vi "READ POV angles.vi"(10 "Buttons":bool[](array[boolean]), 11 "POVs":i16[](array[numeric])) -> ()   [LabVIEW 2020]
uses:
  defCameraPOVservos.ctl
  <vilib>/Analysis/coordinate.llb/Angle Range (Degree).ctl
  <vilib>/Analysis/coordinate.llb/Angle Units.ctl
  <vilib>/Analysis/coordinate.llb/Wrap Angle (scalar).vi
  <vilib>/Rock Robotics/Network Tables/NT Read Number.vi
  <vilib>/Rock Robotics/Network Tables/NT Write Number.vi
  <vilib>/Analysis/NI_AAL_Angle.lvlib
panel:
  in  "CameraServos":cluster{"PAN":T1, "TILT":T1}
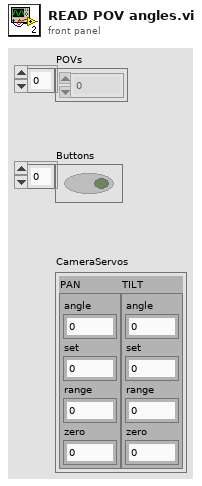
[diagram p1: front panel]
types:
  T1 = typedef "defCameraPOVservos.ctl" = cluster{"angle":dbl, "set":dbl, "range":dbl, "zero":dbl}
  T2 = typedef "NI_AAL_Angle.lvlib/Angle Units.ctl" = i32
  T3 = typedef "NI_AAL_Angle.lvlib/Angle Range (Degree).ctl" = u16
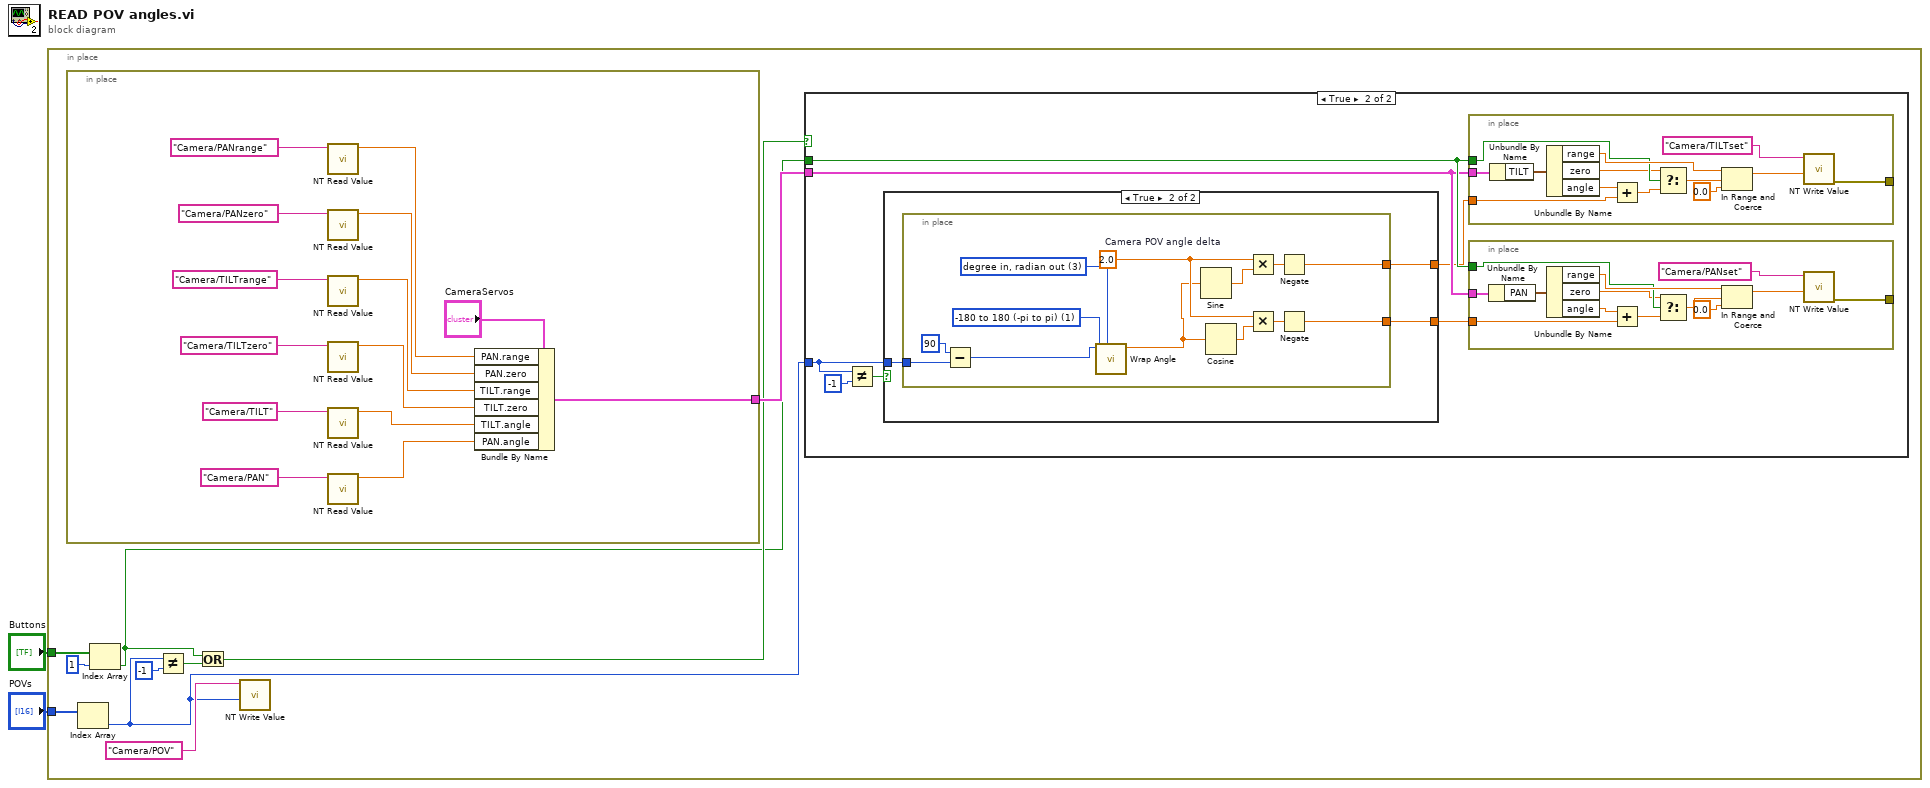
[diagram p0: block diagram]
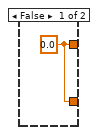
[diagram p3: hidden frame]
diagram:
  n1 = in-place {
    in-place-border: "POVs" -> [w4]
    in-place-border: "Buttons" -> [w3]
    n2 = in-place {
      in-place-border: [w68] -> w12
      n3 = call-poly <vilib>:"NT Read Value.vi"("Name"="Camera/PANrange" ("refnum name")) -> ("Numeric"=w72:dbl)  [unwired: 9 in, 1 out]
      n4 = call-poly <vilib>:"NT Read Value.vi"("Name"="Camera/PANzero" ("refnum name")) -> ("Numeric"=w71:dbl)  [unwired: 9 in, 1 out]
      n5 = call-poly <vilib>:"NT Read Value.vi"("Name"="Camera/TILTrange" ("refnum name")) -> ("Numeric"=w70:dbl)  [unwired: 9 in, 1 out]
      n6 = call-poly <vilib>:"NT Read Value.vi"("Name"="Camera/TILTzero" ("refnum name")) -> ("Numeric"=w69:dbl)  [unwired: 9 in, 1 out]
      n7 = call-poly <vilib>:"NT Read Value.vi"("Name"="Camera/TILT" ("refnum name")) -> ("Numeric"=w65:dbl)  [unwired: 9 in, 1 out]
      n8 = call-poly <vilib>:"NT Read Value.vi"("Name"="Camera/PAN" ("refnum name")) -> ("Numeric"=w64:dbl)  [unwired: 9 in, 1 out]
      n9 = Bundle By Name(cluster="CameraServos", "PAN.range"=w72, "PAN.zero"=w71, "TILT.range"=w70, "TILT.zero"=w69, "TILT.angle"=w65, "PAN.angle"=w64) -> (w68:cluster{"PAN":T1, "TILT":T1})
    }
    n10 = Index Array(array=w4) -> (element=w5:i16)  [unwired: 1 in]
    n11 = Index Array(array=w3, index=1) -> (element=w6:bool)
    n12 = Not Equal?(x=w5, y=i16 -1) -> (x != y?=w10:bool)
    n13 = Or(x=w6, y=w10) -> (x .or. y?=w7:bool)
    n14 = call-poly <vilib>:"NT Write Value.vi"("Numeric"=w5, "Name"="Camera/POV") -> ()  [unwired: 9 in, 1 out]
    n15 = case shown="True" w7 {
      tunnel: w5 -> [_ w14]
      tunnel: w6 -> [_ w19]
      tunnel: w12 -> [_ w18]
      frame False {
      }
      frame True {
        n16 = Not Equal?(x=w14, y=i16 -1) -> (x != y?=w15:bool)
        n17 = case shown="True" w15 {
          tunnel: w14 -> [_ w23]
          tunnel: [w20 w22] -> w17
          tunnel: [w20 w21] -> w16
          frame False {
            w20 = 0.0
          }
          frame True {
            n18 = in-place {
              in-place-border: w23 -> [w30]
              in-place-border: [w35] -> w21
              in-place-border: [w34] -> w22
              w26 = T2 3 items=["radian in, radian out", "radian in, degree out", "degree in, degree out", "degree in, radian out"] ("angle units")
              w27 = T3 1 items=["none", "-180 to 180 (-pi to pi)", "0 to 360 (0 to 2pi)"] ("angle range")
              w33 = 2.0  # Camera POV angle delta
              n19 = Subtract(x=i16 90, y=w30) -> (x-y=w24:i16)
              n20 = call-poly <vilib>:"Wrap Angle.vi"("angle units"=w26, "angle range"=w27, "angle in"=w24) -> ("angle out"=w25:dbl)  [unwired: 7 in, 1 out]
              n21 = Sine(x=w25) -> (sin(x)=w29:dbl)
              n22 = Cosine(x=w25) -> (cos(x)=w28:dbl)
              n23 = Multiply(x=w33, y=w29) -> (x*y=w31:dbl)
              n24 = Multiply(x=w33, y=w28) -> (x*y=w32:dbl)
              n25 = Negate(x=w31) -> (-x=w35:dbl)
              n26 = Negate(x=w32) -> (-x=w34:dbl)
            }
          }
        }
        n27 = in-place {
          in-place-border: w19 -> [w58]
          in-place-border: w18 -> [w51]
          in-place-border: [w55] -> _
          in-place-border: w16 -> [w52]
          n28 = Unbundle By Name(w51) -> ("TILT"=w50:T1)
          n29 = Unbundle By Name(w50) -> ("range"=w59:dbl, "zero"=w57:dbl, "angle"=w54:dbl)
          n30 = Add(x=w54, y=w52) -> (x+y=w53:dbl)
          n31 = Select(t=w57, s=w58, f=w53) -> (s? t:f=w60:dbl)
          n32 = In Range and Coerce(upper limit=w59, x=w60, lower limit=0.0) -> (coerced(x)=w61:dbl)  [unwired: 1 out]
          n33 = call-poly <vilib>:"NT Write Value.vi"("Numeric"=w61, "Name"="Camera/TILTset") -> ("error out"=w55:errorcluster)  [unwired: 9 in]
        }
        n34 = in-place {
          in-place-border: w19 -> [w46]
          in-place-border: w18 -> [w39]
          in-place-border: [w43] -> _
          in-place-border: w17 -> [w40]
          n35 = Unbundle By Name(w39) -> ("PAN"=w38:T1)
          n36 = Unbundle By Name(w38) -> ("range"=w47:dbl, "zero"=w45:dbl, "angle"=w42:dbl)
          n37 = Add(x=w42, y=w40) -> (x+y=w41:dbl)
          n38 = Select(t=w45, s=w46, f=w41) -> (s? t:f=w48:dbl)
          n39 = In Range and Coerce(upper limit=w47, x=w48, lower limit=0.0) -> (coerced(x)=w49:dbl)  [unwired: 1 out]
          n40 = call-poly <vilib>:"NT Write Value.vi"("Numeric"=w49, "Name"="Camera/PANset") -> ("error out"=w43:errorcluster)  [unwired: 9 in]
        }
      }
    }
  }
